vi "ArduinoTester.vi"() -> ()   [LabVIEW 2015]
uses:
  <vilib>/LabVIEW Interface for Arduino/Type Defs/Board Type.ctl
  <vilib>/LabVIEW Interface for Arduino/Type Defs/Connection Type.ctl
  <vilib>/LabVIEW Interface for Arduino/LabVIEW Interface for Arduino.lvlib
panel:
  out "Current Testing":string
  in  "Analog Input Pin (AX)":u8
  in  "Stop Test":bool
  in  "Next":bool
  in  "PWM Pin":u8=3
  out "Voltage":dbl(knob) scale=0.0..5.0
  in  "Duty Cycle (0 - 255)":u8
  # "2. Test Analog Input pins"
  # "1. Test Output of PWM pins"
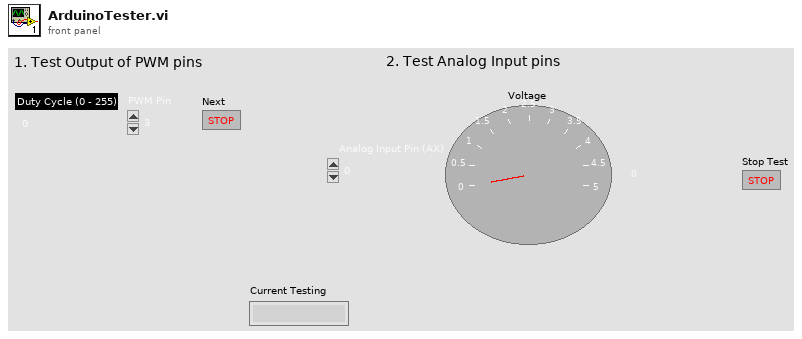
[diagram p1: front panel]
types:
  T1 = typedef "LabVIEW Interface for Arduino.lvlib/Connection Type.ctl" = enum8{"USB / Serial", "XBEE", "BlueSmirf (Bluetooth)"}
  T2 = typedef "LabVIEW Interface for Arduino.lvlib/Board Type.ctl" = enum16{"Uno", "Dimuelanove w/Atmega 328", "Mega 2560"}
  T3 = typedef "LabVIEW Interface for Arduino.lvlib/Arduino Resource.ctl" = cluster{"VISA resource":refnum<visa-resource-name>, "Board Type":T2, "Connection Type":enum8{"USB / Serial"}, "Bytes Per Packet (15)":u8}
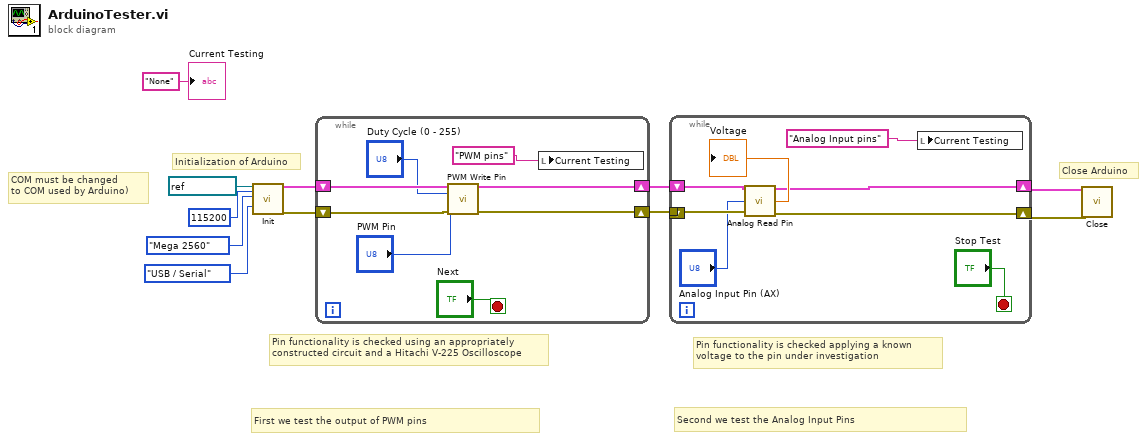
[diagram p0: block diagram]
diagram:
  # "Close Arduino"
  # "Pin functionality is checked applying a known \nvoltage to the pin under investigation"
  # "Second we test the Analog Input Pins"
  # "COM must be changed \nto COM used by Arduino)"
  # "Pin functionality is checked using an appropriately \nconstructed circuit and a Hitachi V-225 Oscilloscope"
  # "Initialization of Arduino"
  # "First we test the output of PWM pins"
  n1 = call <vilib>:"Init.vi"("VISA resource"=refnum<visa-resource-name> "COM10", "Baud Rate (115200)"=u32 115200, "Board Type (Uno)"=Board_Type."Mega 2560", "Connection Type (USB/Serial)"=Connection_Type."USB / Serial") -> ("Arduino Resource"=w7:T3, "error out"=w6:errorcluster)  [unwired: 14 in]
  n2 = while {
    shift-right: [w15] -> w4
    shift-left: w6 -> [w18]
    shift-right: [w16] -> w5
    shift-left: w7 -> [w19]
    stop <- "Next" stop-if-true
    n3 = call <vilib>:"PWM Write Pin.vi"("Arduino Resource"=w19, "Duty Cycle (0 - 255)"="Duty Cycle (0 - 255)", "PWM Pin (3)"="PWM Pin", "error in"=w18) -> ("Arduino Resource"=w16:T3, "error out"=w15:errorcluster)  [unwired: 10 in]
    n4 = local write "Current Testing"("PWM pins" ("Current Testing")) -> ()
  }
  n5 = while {
    tunnel: w4 -> [w26]
    shift-right: [w23] -> w3
    shift-left: w5 -> [w27]
    shift-right: [w24] -> w2
    shift-left: _ -> [_]
    stop <- "Stop Test" stop-if-true
    n6 = call <vilib>:"Analog Read Pin.vi"("Arduino Resource"=w27, "Analog Input Pin (0)"="Analog Input Pin (AX)", "error in"=w26) -> ("Arduino Resource"=w23:T3, "Voltage"=→"Voltage":dbl, "error out"=w24:errorcluster)  [unwired: 10 in]
    n7 = local write "Current Testing"("Analog Input pins" ("Current Testing")) -> ()
  }
  n8 = call <vilib>:"Close.vi"("Arduino Resource"=w3, "error in"=w2) -> ()  [unwired: 13 in, 1 out]
  "Current Testing" <- "None" ("Current Testing")
